vi "MtAtElectrometer_logEvent_intensity.vi"(8 "error in (no error)":errorcluster, 11 "logevent_intensity_Ctl":T1) -> (0 "error out":errorcluster, 2 "function return":i32, 3 "logevent_intensity_Ctl out":T1)   [LabVIEW 2016, in "SALLV_MtAtElectrometer.lvlib"]
doc: "int MtAtElectrometer_shm_logEvent_intensityLV(MtAtElectrometer_logevent_intensityLV *logevent_intensity_Ctl );"
uses:
  SALLV_MtAtElectrometer.lvlib
  DataTypes/logevent_intensity.ctl
  ts_sal/test/MtAtElectrometer/labview/SALLV_MtAtElectrometer.so
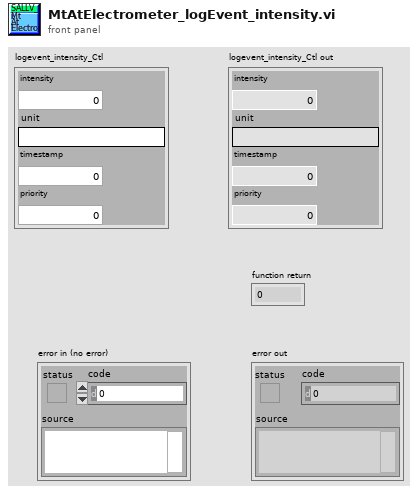
[diagram p1: front panel]
types:
  T1 = typedef "SALLV_MtAtElectrometer.lvlib/logevent_intensity.ctl" = cluster{"intensity":dbl, "unit":string, "timestamp":dbl, "priority":i32}
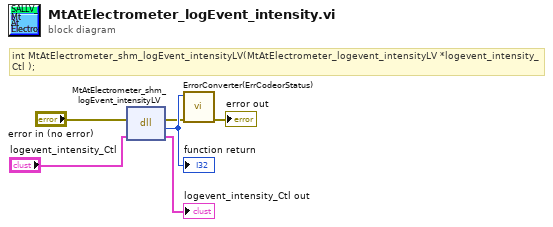
[diagram p0: block diagram]
diagram:
  # "int MtAtElectrometer_shm_logEvent_intensityLV(MtAtElectrometer_logevent_intensityLV *logevent_intensity_Ctl );"
  n1 = dll-call lib="home/andres/ts_sal/test/MtAtElectrometer/labview/SALLV_MtAtElectrometer.*" fn="MtAtElectrometer_shm_logEvent_intensityLV"(error in="error in (no error)", "logevent_intensity_Ctl"="logevent_intensity_Ctl") -> (error out=w2:errorcluster, w6:i32, "logevent_intensity_Ctl"=→"logevent_intensity_Ctl out":T1)  [unwired: 2 in, 1 out]
  "function return" <- w6
  n2 = call "ErrorConverter(ErrCodeorStatus).vi"("error in (no error)"=w2, "error code"=w6) -> ("error out"=→"error out":errorcluster)  [unwired: 9 in]
